vi "corrello.vi"() -> ()   [LabVIEW 2010]
uses:
  <vilib>/ptbypt/NI_PtbyPt.lvlib
panel:
  out "subarray":dbl[](array[numeric])
  out "max index(es)":i32
  out "max value":dbl
  out "y":dbl[](graph)
  out "x":dbl[](graph)
  in  "stop 2":bool
  out "Array 2":dbl[](array[numeric])
  out "Array":dbl[](array[numeric])
  out "cross correlation":dbl[](graph)
  out "Rxy":dbl[](array[numeric])
  in  "stop":bool
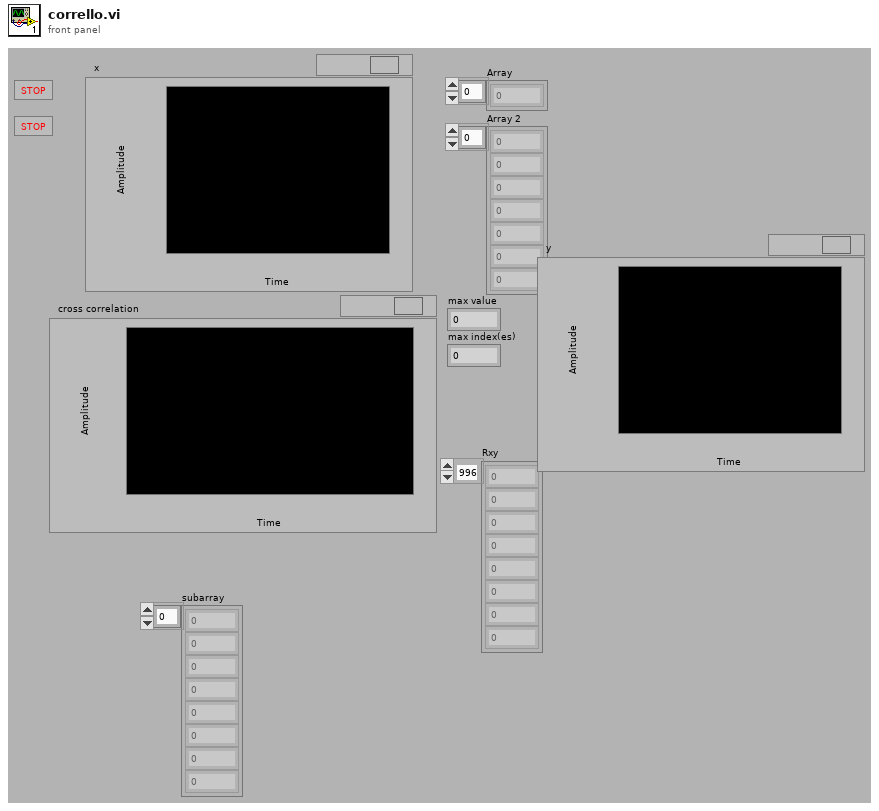
[diagram p1: front panel]
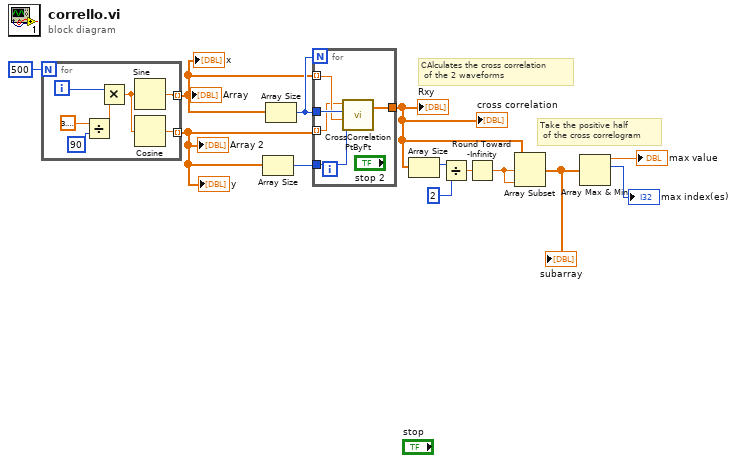
[diagram p0: block diagram]
diagram:
  # "Take the positive half\n of the cross correlogram"
  # "CAlculates the cross correlation\n of the 2 waveforms"
  n1 = for {
    N: 500 -> [_]
    tunnel: [w16] -> w9 mode=indexing
    tunnel: [w15] -> w10 mode=indexing
    i -> [w14]
    n2 = Divide(x=3.141592653589793, y=90) -> (x/y=w18:dbl)
    n3 = Multiply(x=w14, y=w18) -> (x*y=w17:dbl)
    n4 = Sine(x=w17) -> (sin(x)=w16:dbl)
    n5 = Cosine(x=w17) -> (cos(x)=w15:dbl)
  }
  "Array" <- w9
  "Array 2" <- w10
  "x" <- w9
  "y" <- w10
  n6 = Array Size(array=w10) -> (size(s)=w12:i32)
  n7 = Array Size(array=w9) -> (size(s)=w11:i32)
  n8 = for {
    N: w11 -> [_]
    tunnel: [w25] -> w3
    tunnel: w11 -> [w24]
    tunnel: w12 -> [w23]
    tunnel: w9 -> [w22] mode=indexing
    tunnel: w10 -> [w21] mode=indexing
    n9 = call <vilib>:"CrossCorrelation PtByPt.vi"("x"=w21, "sample length x"=w24, "y"=w22, "sample length y"=w23) -> ("Rxy"=w25:dbl[])  [unwired: 1 in, 1 out]
  }
  "Rxy" <- w3
  "cross correlation" <- w3
  n10 = Array Size(array=w3) -> (size(s)=w8:i32)
  n11 = Divide(x=w8, y=2) -> (x/y=w2:dbl)
  n12 = Round Toward -Infinity(1:w2) -> (0:w7:dbl)
  n13 = Array Subset(array=w3, index=w7, length=w7) -> (w6:dbl[])
  "subarray" <- w6
  n14 = Array Max & Min(array=w6) -> (max value=→"max value":dbl, max index (indices)=→"max index(es)":i32)  [unwired: 2 out]
